vi "TrapProfile_New.vi"(9 "Initial":T1 {"Velocity" format="%16_6e"; "Position" format="%16_6e"}, 10 "Goal":T1 {"Velocity" format="%16_6e"; "Position" format="%16_6e"}, 11 "Constraints":T2 {"MaxAcceleration" format="%16_6e"; "MaxVelocity" format="%16_6e"}) -> (3 "TRAPEZOID_PROFILE":T3 {"Goal"."Velocity" format="%16_6e"; "Goal"."Position" format="%16_6e"; "Initial"."Velocity" format="%16_6e"; "Initial"."Position" format="%16_6e"; "Constraints"."MaxAcceleration" format="%16_6e"; "Constraints"."MaxVelocity" format="%16_6e"; "EndDecel" format="%16_6e"; "EndFullSpeed" format="%16_6e"; "EndAccel" format="%16_6e"})   [LabVIEW 2019, in "Trajectory_Library.lvlib"]
doc: "Construct a TrapezoidProfile data cluster and performs initial calculations to fill data cluster\n \nInputs:\n - constraints -- The constraints on the profile, like maximum velocity.\n - goal -- The desired state when the profile is complete.\n - initial -- The initial state (usually the current state).\n\nOutputs:\n - Trapezoid_Profile -- Initialized Trapezoid_Profile data cluster"
uses:
  Trajectory_Library.lvlib
  TRAPEZOID_PROFILE.ctl
  TRAPEZOID_PROFILE_CONSTRAINT.ctl
  TRAPEZOID_PROFILE_STATE.ctl
  TrapProfState_New.vi
  <vilib>/Rock Robotics/SystemInterfaces/NetworkCommunication/NetComm_UsageReport_ResourceType.ctl
  Util_LibraryGlobals.vi
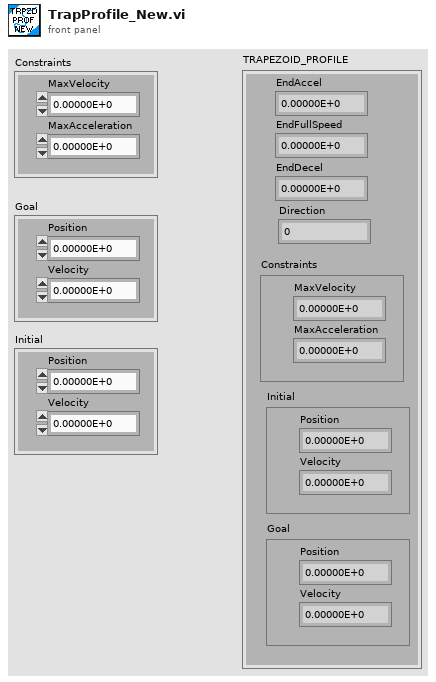
[diagram p1: front panel]
types:
  T1 = typedef "Trajectory_Library.lvlib/TRAPEZOID_PROFILE_STATE.ctl" = cluster{"Position":dbl, "Velocity":dbl}
  T2 = typedef "Trajectory_Library.lvlib/TRAPEZOID_PROFILE_CONSTRAINT.ctl" = cluster{"MaxVelocity":dbl, "MaxAcceleration":dbl}
  T3 = typedef "Trajectory_Library.lvlib/TRAPEZOID_PROFILE.ctl" = cluster{"EndAccel":dbl, "EndFullSpeed":dbl, "EndDecel":dbl, "Direction":i32, "Constraints":T2, "Initial":T1, "Goal":T1}
  T4 = typedef "NetComm_UsageReport_ResourceType.ctl" = enum8{"Controller", "Module", "Language", "CANPlugin", "Accelerometer", "ADXL345", "AnalogChannel", "AnalogTrigger", "AnalogTriggerOutput", "CANJaguar", "Compressor", "Counter", "Dashboard", "DigitalInput", "DigitalOutput", "DriverStationCIO", "DriverStationEIO", "DriverStationLCD", "Encoder", "GearTooth", "Gyro", "I2C", "Framework", "Jaguar", "Joystick", "Kinect", "KinectStick", "PIDController", "Preferences", "PWM", "Relay", "RobotDrive", "SerialPort", "Servo", "Solenoid", "SPI", "Task", "Ultrasonic", "Victor", "Button", "Command", "AxisCamera", "PCVideoServer", "SmartDashboard", "Talon", "HiTechnicColorSensor", "HiTechnicAccel", "HiTechnicCompass", "SRF08", "AnalogOutput", "Victor SP", "Talon SRX", "CAN Talon SRX", "ADXL362 Accel", "ADXRS450 Gyro", "Rev SPARK", "Mindsensors SD540", "Digital Filter", "ADIS16448", "PDP", "PCM", "PigeonIMU", "Nidec Brushless", "CTRE CANifier", "CTRE TalonFX", "CTRE Future 1", "CTRE Future 2", "CTRE Future 3", "CTRE Future 4", "CTRE Future 5", "CTRE Future 6", "Linear Filter", "Xbox Controller", "USB Camera", "NavX", "Pixy", "Pixy2", "ScanseSweep", "Shuffleboard", "CAN", "Digilent DMC60", "PWM Victor SPX", "Rev SPARK MAX PWM", "Rev SPARK MAX CAN", "ADIS16470", "PIDController2", "ProfiledPIDController", "Kinematics", "Odometry", "Units", "Trapezoid Profile", "DutyCycle", "Addressable LEDs", "Fusion Venom"}
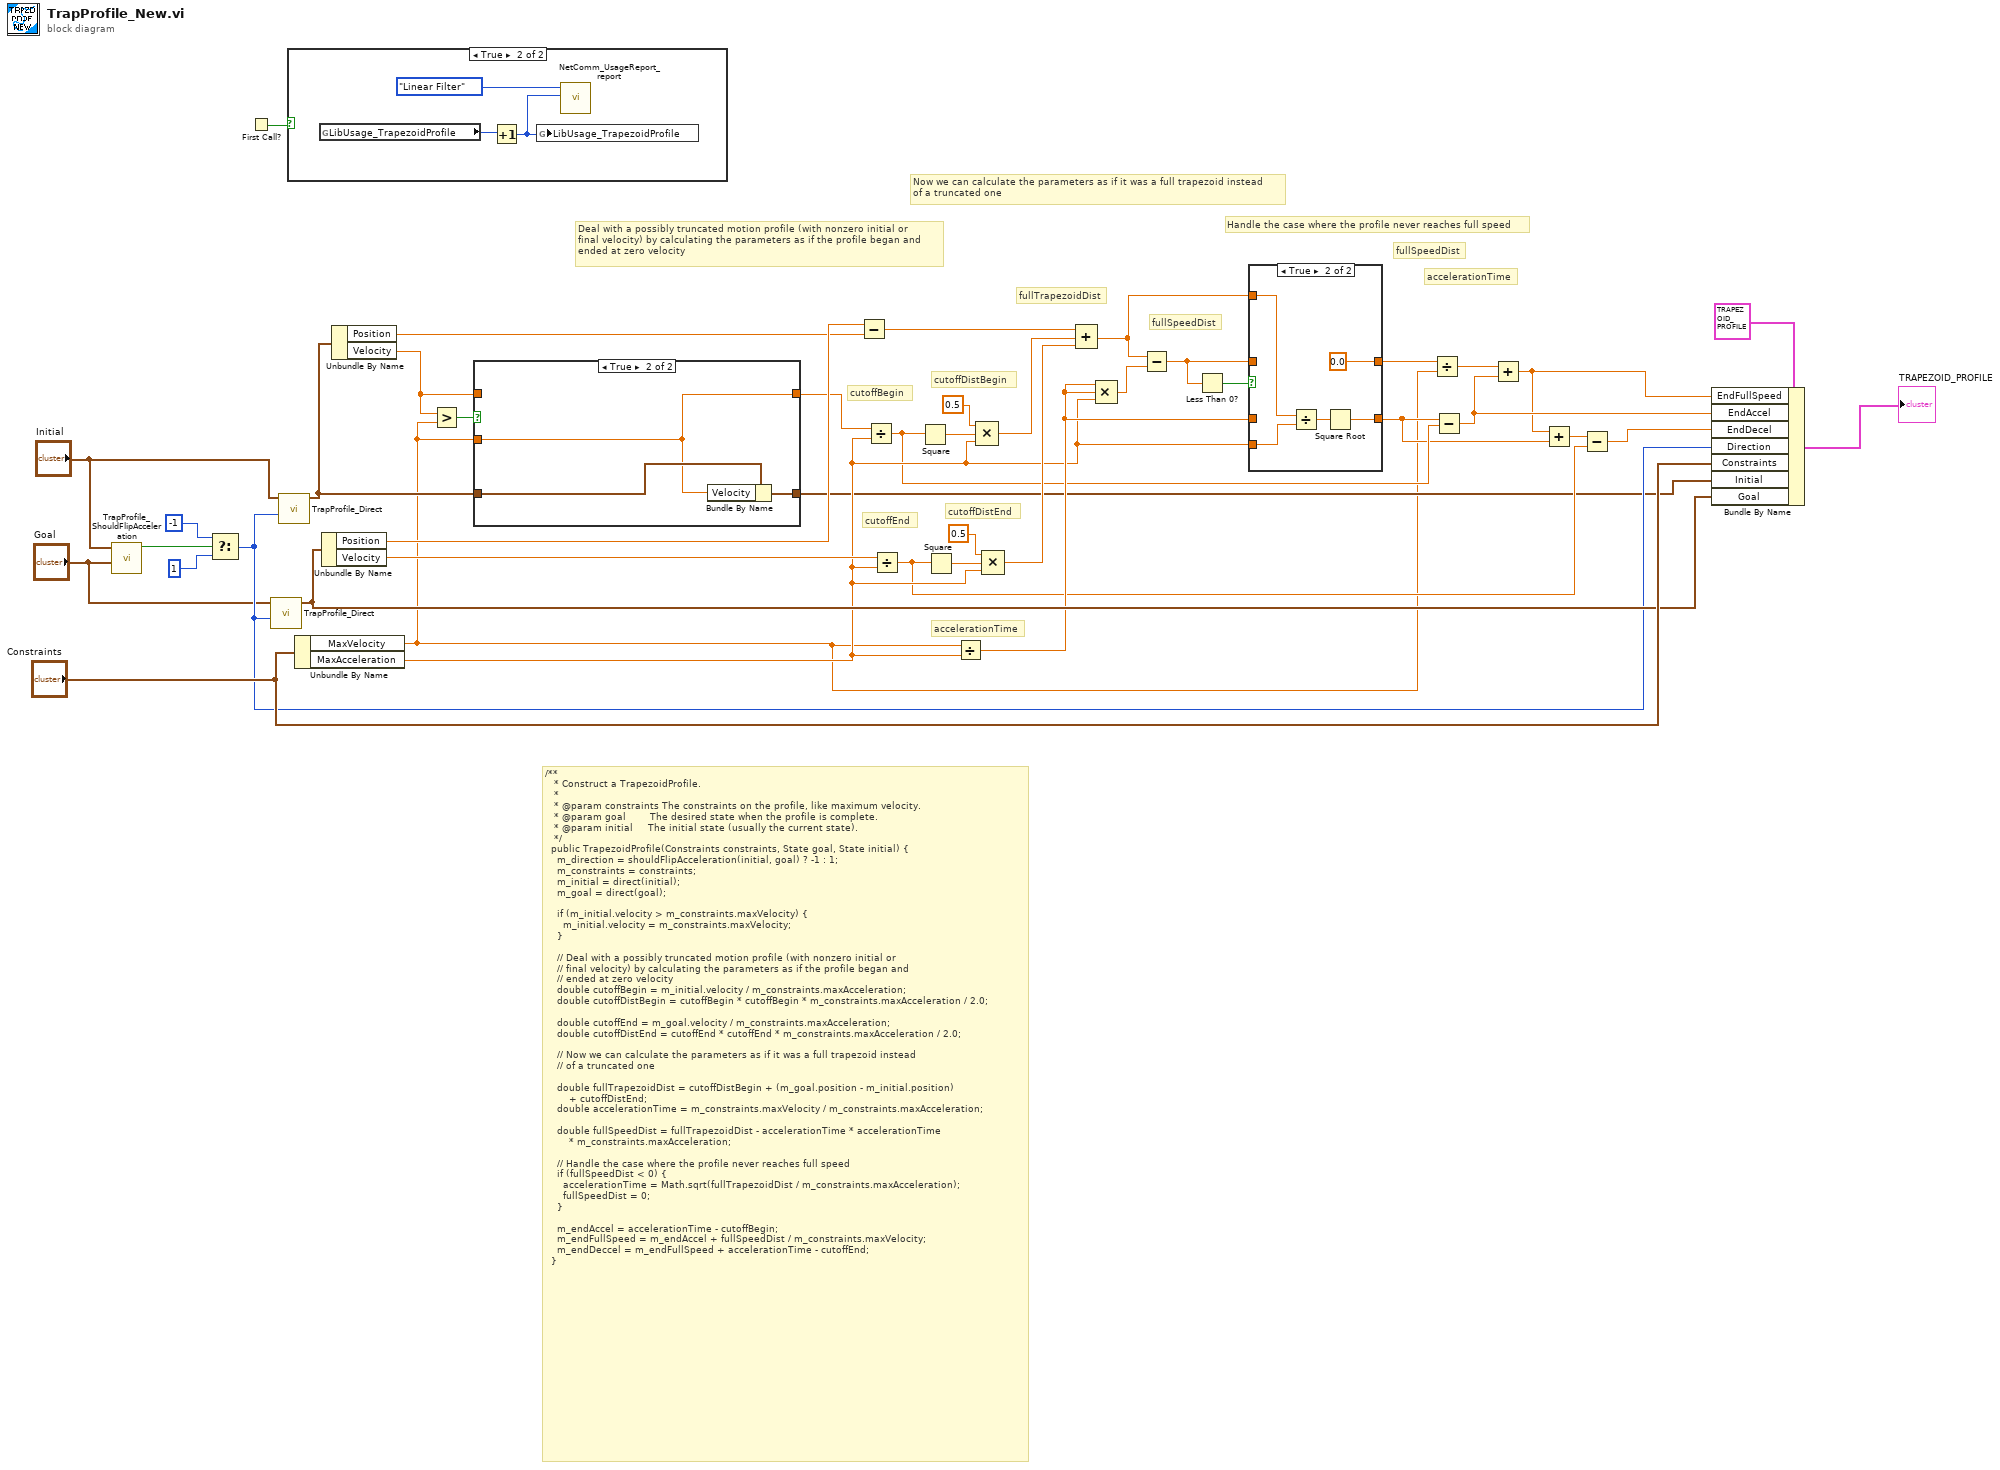
[diagram p0: block diagram]
diagram:
  # "Handle the case where the profile never reaches full speed"
  # "Now we can calculate the parameters as if it was a full trapezoid instead\nof a truncated one"
  # "Deal with a possibly truncated motion profile (with nonzero initial or\nfinal velocity) by calculating the parameters as if the profile began and\nended at zero velocity"
  # "accelerationTime"
  # "fullSpeedDist"
  # "fullSpeedDist"
  # "accelerationTime"
  # "fullTrapezoidDist"
  # "cutoffDistEnd"
  # "cutoffEnd"
  # "cutoffDistBegin"
  # "cutoffBegin"
  # "/**\n   * Construct a TrapezoidProfile.\n   *\n   * @param constraints The constraints on the profile, like maximum velocity.\n   * @param goal        The desired state when the profile is complete.\n   * @param initial     The initial state (usually the current state).\n   */\n  public TrapezoidProfile(Constraints constraints, State goal, State initial) {\n    m_direction = shouldFlipAcceleration(initial, goal) ? -1 : 1;\n    m_constraints = constraints;\n    m_initial = direct(initial);\n    m_goal = direct(goal);\n\n    if (m_initial.velocity > m_constraints.maxVelocity) {\n      m_initial.velocity = m_constraints.maxVelocity;\n    }\n\n    // Deal with a possibly truncated motion profile (with nonzero initial or\n    // final velocity) by calculating the parameters as if the profile began and\n    // ended at zero velocity\n    double cutoffBegin = m_initial.velocity / m_constraints.maxAcceleration;\n    double cutoffDistBegin = cutoffBegin * cutoffBegin * m_constraints.maxAcceleration / 2.0;\n\n    double cutoffEnd = m_goal.velocity / m_constraints.maxAcceleration;\n    double cutoffDistEnd = cutoffEnd * cutoffEnd * m_constraints.maxAcceleration / 2.0;\n\n    // Now we can calculate the parameters as if it was a full trapezoid instead\n    // of a truncated one\n\n    double fullTrapezoidDist = cutoffDistBegin + (m_goal.position - m_initial.position)\n        + cutoffDistEnd;\n    double accelerationTime = m_constraints.maxVelocity / m_constraints.maxAcceleration;\n\n    double fullSpeedDist = fullTrapezoidDist - accelerationTime * accelerationTime\n        * m_constraints.maxAcceleration;\n\n    // Handle the case where the profile never reaches full speed\n    if (fullSpeedDist < 0) {\n      accelerationTime = Math.sqrt(fullTrapezoidDist / m_constraints.maxAcceleration);\n      fullSpeedDist = 0;\n    }\n\n    m_endAccel = accelerationTime - cutoffBegin;\n    m_endFullSpeed = m_endAccel + fullSpeedDist / m_constraints.maxVelocity;\n    m_endDeccel = m_endFullSpeed + accelerationTime - cutoffEnd;\n  }"
  n1 = call "TrapProfile_ShouldFlipAcceleration.vi"("goal TRAPEZOID_PROFILE_STATE"="Goal", "Initial TRAPEZOID_PROFILE_STATE"="Initial") -> ("Flip"=w38:bool)  [unwired: 9 in]
  n2 = Select(t=-1, s=w38, f=1) -> (s? t:f=w9:i32)
  n3 = First Call?() -> (First Call?: T/F=w1:bool)
  n4 = call "TrapProfile_Direct.vi"("Direction"=w9, "in TRAPEZOID_PROFILE_STATE"="Goal") -> ("out TRAPEZOID_PROFILE_STATE"=w32:T1)  [unwired: 9 in]
  n5 = call "TrapProfile_Direct.vi"("Direction"=w9, "in TRAPEZOID_PROFILE_STATE"="Initial") -> ("out TRAPEZOID_PROFILE_STATE"=w4:T1)  [unwired: 9 in]
  n6 = case shown="True" w1 {
    frame False {
    }
    frame True {
      n7 = global read "Util_LibraryGlobals.vi" "LibUsage_TrapezoidProfile"() -> (w44:i32)
      n8 = Increment(x=w44) -> (x+1=w43:i32)
      n9 = global write "Util_LibraryGlobals.vi" "LibUsage_TrapezoidProfile"(w43) -> ()
      n10 = call <vilib>:"NetComm_UsageReport_report.vi"("Instance Number"=w43, "Resource Type"=NetComm_UsageReport_ResourceType."Linear Filter") -> ()  [unwired: 10 in]
    }
  }
  n11 = Unbundle By Name("Constraints") -> ("MaxVelocity"=w2:dbl, "MaxAcceleration"=w20:dbl)
  n12 = Unbundle By Name(w32) -> ("Position"=w30:dbl, "Velocity"=w31:dbl)
  n13 = Unbundle By Name(w4) -> ("Position"=w29:dbl, "Velocity"=w5:dbl)
  n14 = Greater?(x=w5, y=w2) -> (0:w6:bool)
  n15 = case shown="True" w6 {
    tunnel: w5 -> [w47 _]
    tunnel: [w47 w48] -> w7
    tunnel: w4 -> [w46 w50]
    tunnel: [w46 w49] -> w3
    tunnel: w2 -> [_ w48]
    frame False {
    }
    frame True {
      n16 = Bundle By Name(cluster=w50, "Velocity"=w48) -> (w49:T1)
    }
  }
  n17 = Subtract(x=w30, y=w29) -> (x-y=w26:dbl)
  n18 = Divide(x=w7, y=w20) -> (x/y=w19:dbl)
  n19 = Divide(x=w31, y=w20) -> (x/y=w11:dbl)
  n20 = Square(x=w19) -> (x^2=w36:dbl)
  n21 = Square(x=w11) -> (x^2=w34:dbl)
  n22 = Divide(x=w2, y=w20) -> (x/y=w21:dbl)
  n23 = Compound Arithmetic op=MULTIPLY(0.5 ("value"), w36, w20) -> (w28:dbl)
  n24 = Compound Arithmetic op=MULTIPLY(0.5 ("value"), w34, w20) -> (w27:dbl)
  n25 = Compound Arithmetic op=ADD(w26, w28, w27) -> (w22:dbl)
  n26 = Compound Arithmetic op=MULTIPLY(w21, w21, w20) -> (w25:dbl)
  n27 = Subtract(x=w22, y=w25) -> (x-y=w23:dbl)
  n28 = Less Than 0?(x=w23) -> (x < 0?=w24:bool)
  n29 = case shown="True" w24 {
    tunnel: w23 -> [w52 _]
    tunnel: [w52 0.0] -> w18
    tunnel: w22 -> [_ w54]
    tunnel: w21 -> [w51 _]
    tunnel: w20 -> [_ w53]
    tunnel: [w51 w56] -> w13
    frame False {
    }
    frame True {
      n30 = Divide(x=w54, y=w53) -> (x/y=w55:dbl)
      n31 = Square Root(x=w55) -> (sqrt(x)=w56:dbl)
    }
  }
  n32 = Divide(x=w18, y=w2) -> (x/y=w16:dbl)
  n33 = Subtract(x=w13, y=w19) -> (x-y=w17:dbl)
  n34 = Add(x=w16, y=w17) -> (x+y=w14:dbl)
  n35 = Add(x=w14, y=w13) -> (x+y=w15:dbl)
  n36 = Subtract(x=w15, y=w11) -> (x-y=w12:dbl)
  n37 = Bundle By Name(cluster=T3 {"EndAccel"=0.0, "EndFullSpeed"=0.0, "EndDecel"=0.0, "Direction"=0, "Constraints"={"MaxVelocity"=0.0, "MaxAcceleration"=0.0}, "Initial"={"Position"=0.0, "Velocity"=0.0}, "Goal"={"Position"=0.0, "Velocity"=0.0}} ("TRAPEZOID_PROFILE"), "EndFullSpeed"=w14, "EndAccel"=w17, "EndDecel"=w12, "Direction"=w9, "Constraints"="Constraints", "Initial"=w3, "Goal"=w32) -> (→"TRAPEZOID_PROFILE":T3)
